vi "TCL.vi"() -> ()   [LabVIEW 2019]
uses:
  TPS Global.vi
panel:
  out "folder_base_2":path
  out "file_name_2":string
  out "file_basename_2":string
  out "time_string_2":string
  out "nfs_ok_2":bool
  out "nfs_ok":bool
  out "nfs_path":path
  out "signal_names":string[](array[string])
  out "time_string":string
  out "file_basename":string
  out "file_name":string
  out "folder_base":path
  in  "nfs_folder":string="z:\\e1039_data\\target_data\\NMR"
  out "discarded fragments":string[](array[string])
  out "signals":cluster{"name":string, "values":string[]}[](array[cluster])
  out "events (last 11)":string[][](array[string])
  out "fragments":string[](array[string])
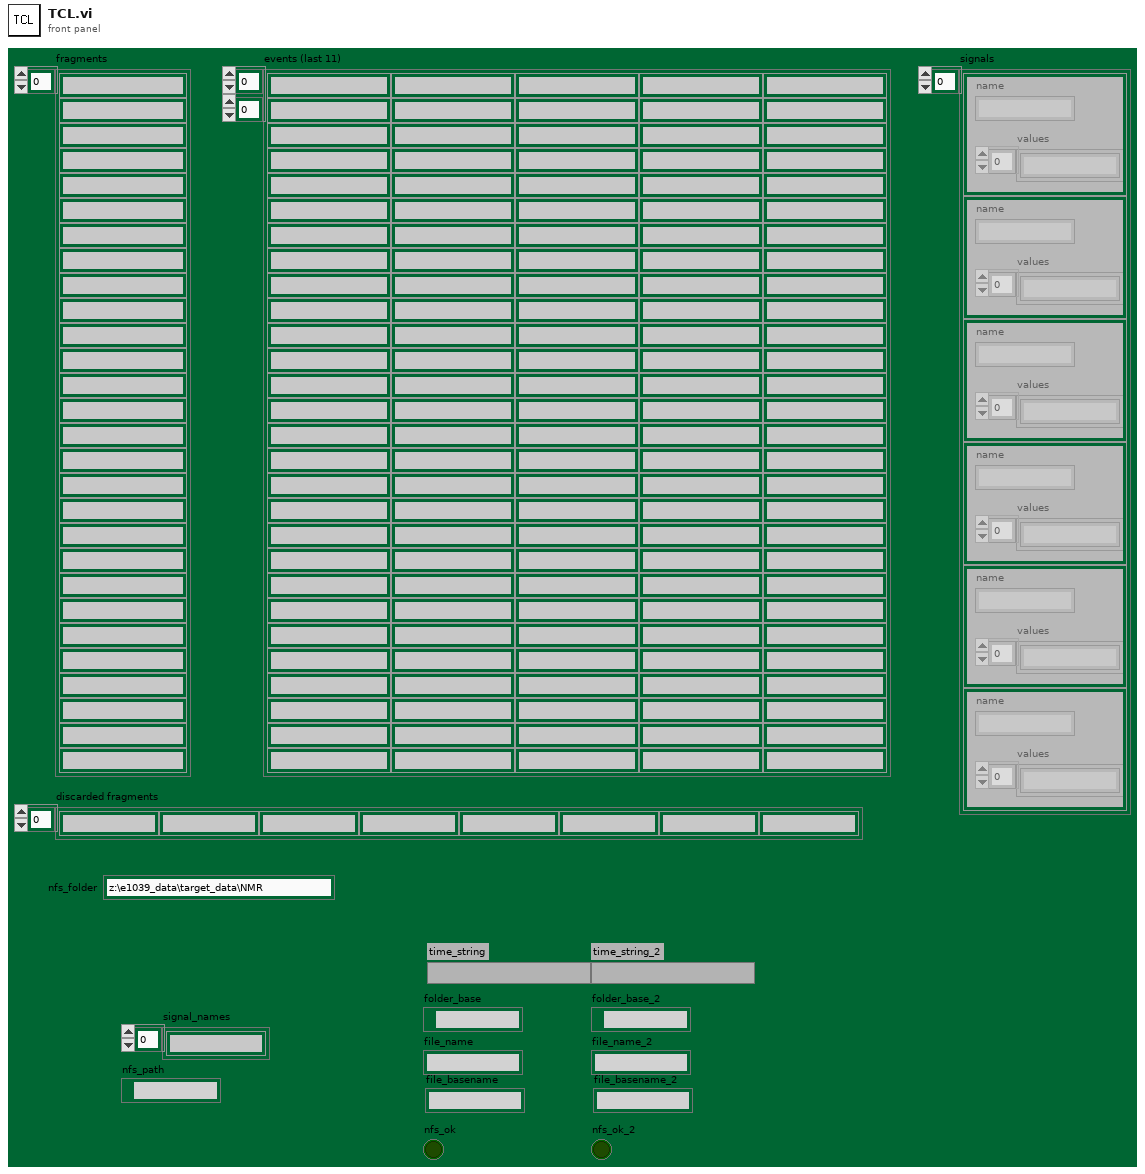
[diagram p1: front panel]
types:
  T1 = enum16{"open", "replace", "create", "open or create", "replace or create", "replace or create with confirmation"}
  T2 = enum16{"No Message", "Bad Message", "NewEventFile", "NewBaseFile", "Event=", "Ping=", "Address=", "Stop"}
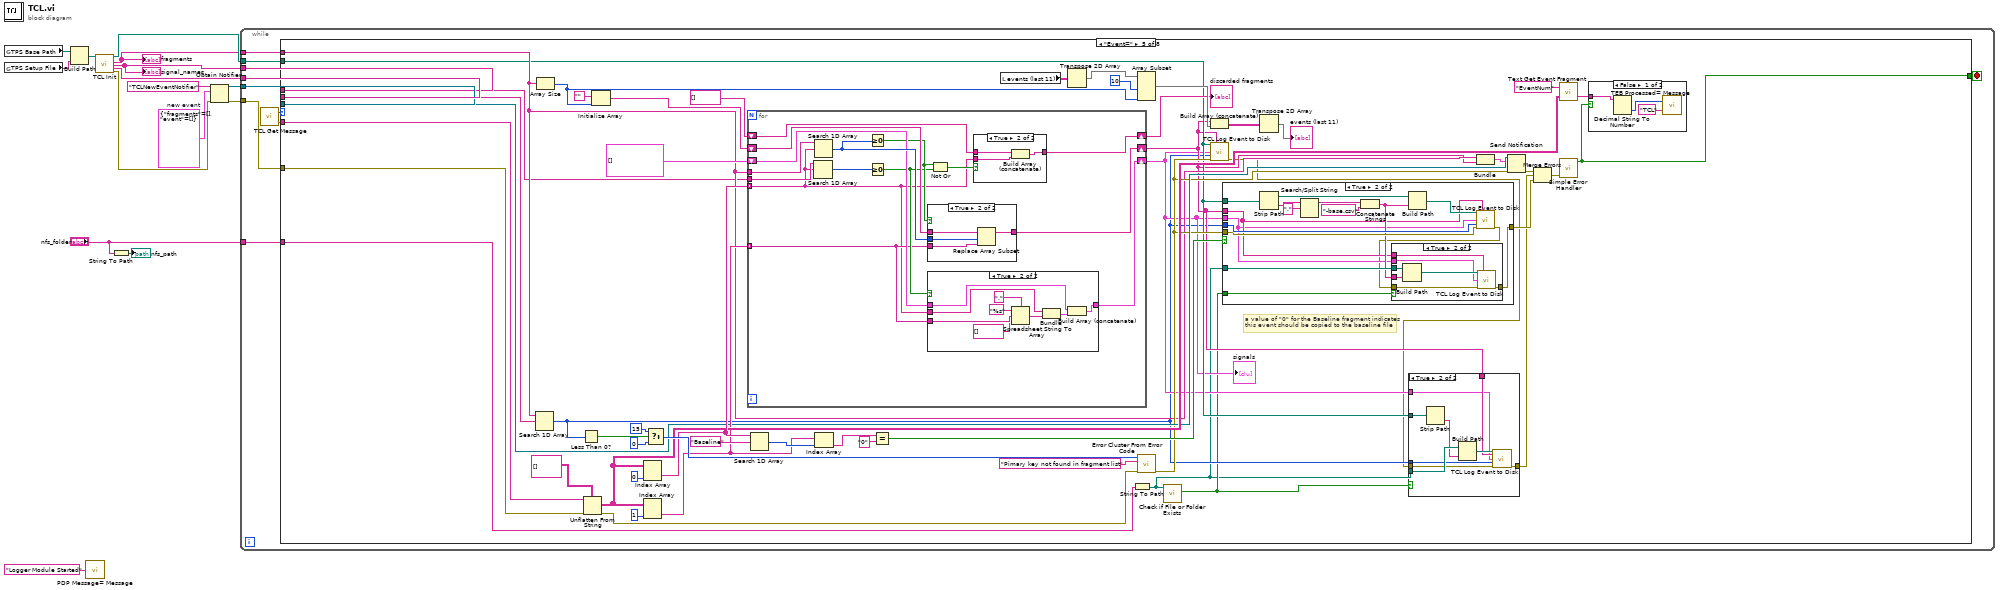
[diagram p0: block diagram]
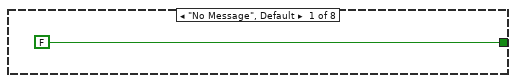
[diagram p2: hidden frame]
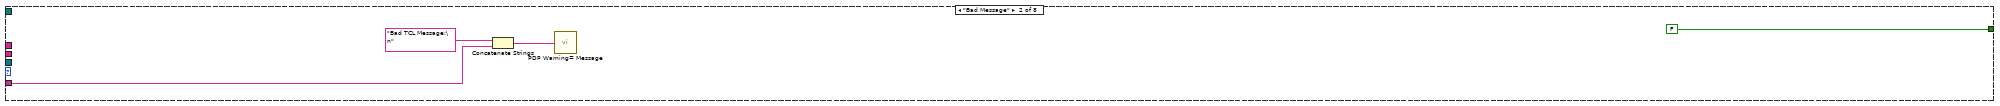
[diagram p3: hidden frame]
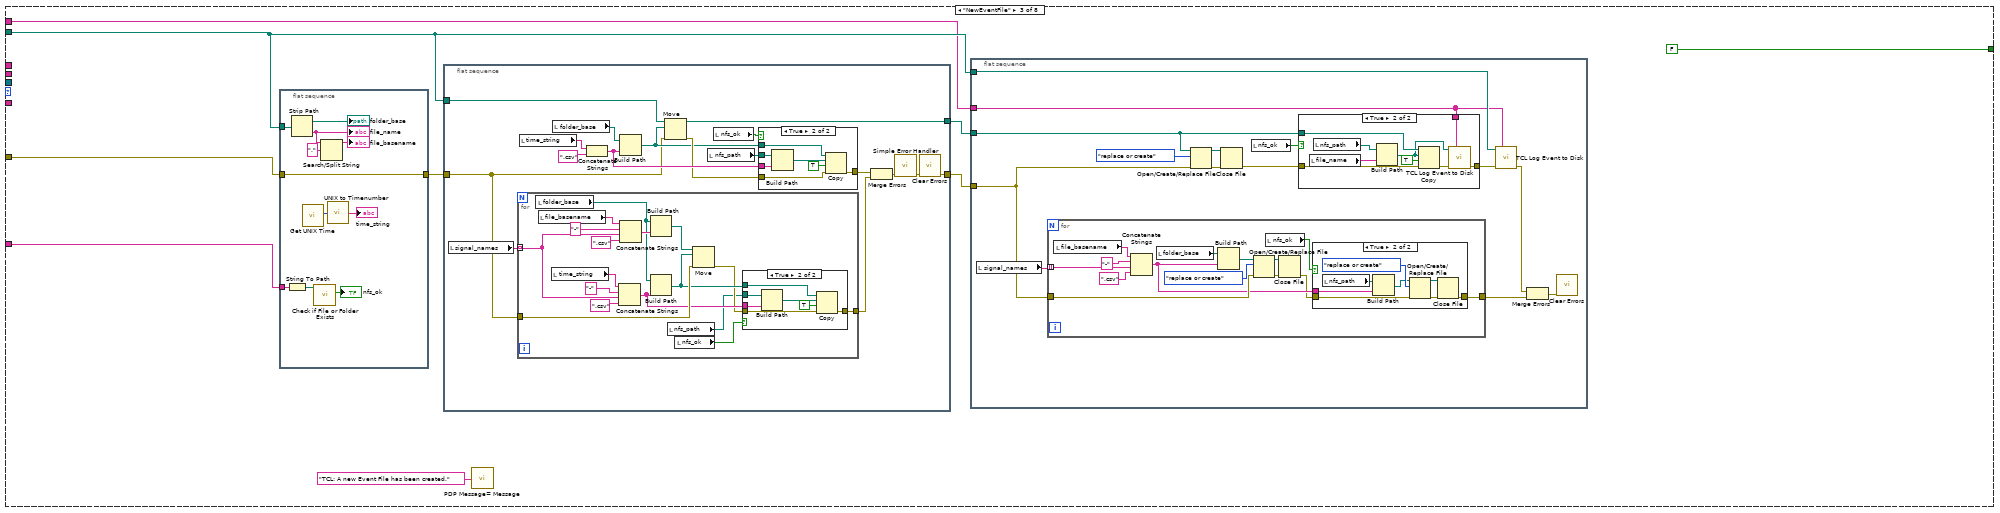
[diagram p4: hidden frame]
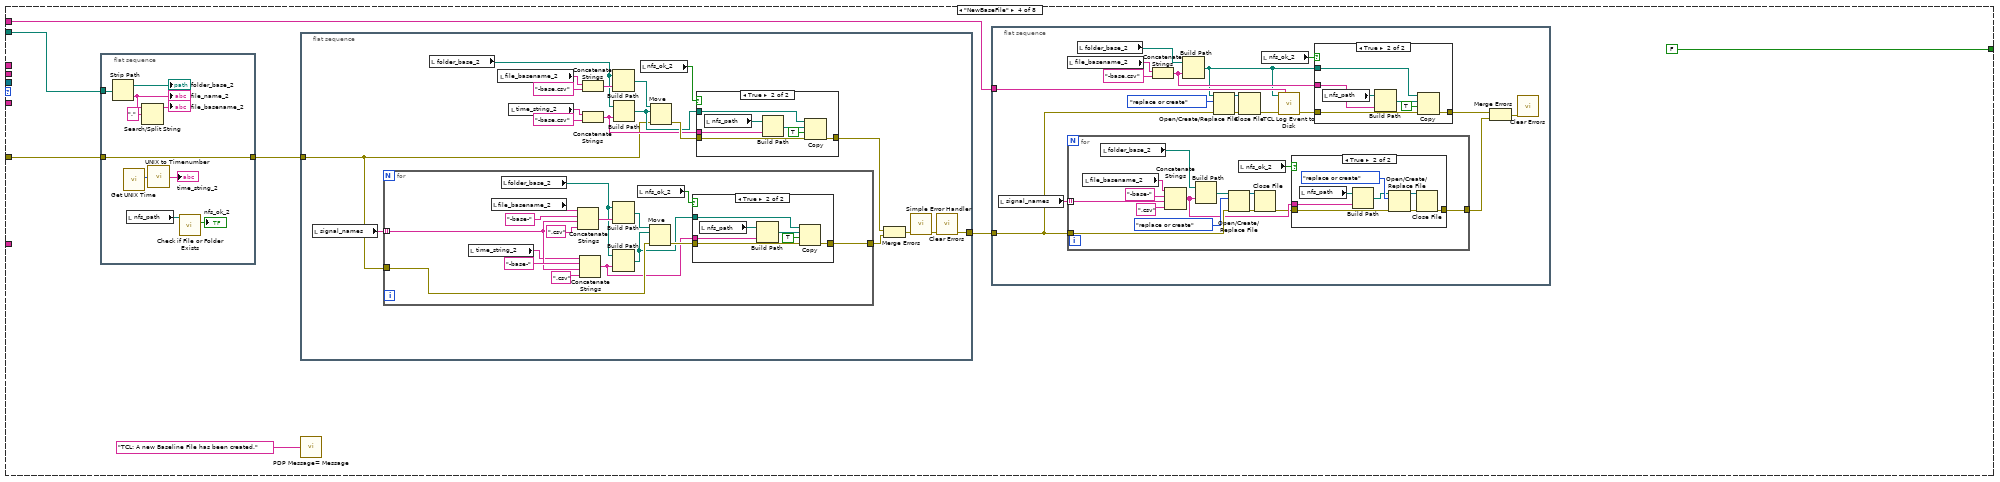
[diagram p9: hidden frame]
diagram:
  w6 = cluster{"fragments":string[], "event":string[]} {"fragments"=[], "event"=[]}  # new event
  n1 = global read "TPS Global.vi" "TPS Base Path"() -> (w14:path)
  n2 = global read "TPS Global.vi" "TPS Setup File"() -> (w13:string)
  n3 = Build Path(base path=w14, name or relative path=w13) -> (appended path=w12:path)
  n4 = call "PDP Message= Message.vi"("Message"="Logger Module Started") -> ()
  n5 = call "TCL Init.vi"("config file"=w12) -> ("event file"=w11:path, "fragments"=w9:string[], "signals"=w3:string[], "primary key"=w10:string, "error out"=w7:errorcluster)  [unwired: 14 in]
  "fragments" <- w9
  "signal_names" <- w3
  n6 = String To Path(string="nfs_folder") -> (path=→"nfs_path":path)
  n7 = Obtain Notifier(name (unnamed)="TCLNewEventNotifier", notification data type=w6, error in (no error)=w7) -> (notifier out=w4:refnum<notifier>, error out=w8:errorcluster)  [unwired: 1 in, 1 out]
  n8 = while {
    tunnel: w8 -> [w23]
    tunnel: w11 -> [w22]
    tunnel: w9 -> [w21]
    tunnel: w10 -> [w19]
    tunnel: w4 -> [w18]
    tunnel: "nfs_folder" -> [w17]
    tunnel: w3 -> [w16]
    stop <- w20 stop-if-true
    n9 = call "TCL Get Message.vi"() -> ("Text"=w24:string, "TCL Message Type"=w25:T2)
    n10 = case shown="\"Event=\"" w25 {
      tunnel: w24 -> [_ w28 _ _ w312 w387 w393 _]
      tunnel: w23 -> [_ _ w34 w148 w313 _ _ _]
      tunnel: w22 -> [_ _ w32 w149 w270 _ _ _]
      tunnel: w21 -> [_ _ w31 w151 w272 _ _ _]
      tunnel: [FALSE FALSE FALSE FALSE w278 FALSE FALSE TRUE] -> w20
      tunnel: w19 -> [_ _ _ _ w304 _ _ _]
      tunnel: w18 -> [_ _ _ _ w276 _ _ _]
      tunnel: w17 -> [_ _ w36 _ w271 _ _ _]
      tunnel: w16 -> [_ _ _ _ w264 _ _ _]
      frame "No Message", Default {
      }
      frame "Bad Message" {
        n11 = Concatenate Strings("Bad TCL Message:\n" ("Message"), w28) -> (w29:string)
        n12 = call "PDP Warning= Message.vi"("Message"=w29) -> ()
      }
      frame "NewEventFile" {
        n13 = flat-sequence {
          tunnel: w36 -> [w144]
          tunnel: w32 -> [w142]
          tunnel: w34 -> [w136]
          tunnel: [w136] -> w33
          frame #0 {
            n14 = String To Path(string=w144) -> (path=w137:path)
            n15 = Strip Path(path=w142) -> (stripped path=→"folder_base":path, name=w140:string)
            "file_name" <- w140
            n16 = call "Get UNIX Time.vi"() -> ("UNIX seconds"=w146:i32)  [unwired: 10 in, 1 out]
            n17 = call <vilib>:"Check if File or Folder Exists.vi"("path"=w137) -> ("file or folder exists?"=→"nfs_ok":bool)  [unwired: 8 in, 2 out]
            n18 = Search/Split String(string=w140, search string/char (-)=".") -> (substring before match=→"file_basename":string)  [unwired: 1 in, 2 out]
            n19 = call "UNIX to Timenumber.vi"("Seconds"=w146) -> ("Timestamp String"=→"time_string":string)
          }
        }
        n20 = flat-sequence {
          tunnel: [w98] -> w37
          tunnel: [w87] -> w35
          tunnel: w33 -> [w88]
          tunnel: w32 -> [w87]
          frame #0 {
            n21 = local read "signal_names"() -> (w93:string[])
            n22 = for {
              tunnel: w93 -> [w121] mode=indexing
              tunnel: w88 -> [w127]
              tunnel: [w116] -> w101
              n23 = local read "folder_base"() -> (w113:path)
              n24 = local read "file_basename"() -> (w114:string)
              n25 = local read "time_string"() -> (w115:string)
              n26 = Concatenate Strings(w115, "-" ("string"), w121, ".csv" ("string")) -> (w119:string)
              n27 = Concatenate Strings(w114, "-" ("string"), w121, ".csv" ("string")) -> (w126:string)
              n28 = Build Path(base path=w113, name or relative path=w126) -> (appended path=w123:path)
              n29 = Build Path(base path=w113, name or relative path=w119) -> (appended path=w118:path)
              n30 = local read "nfs_path"() -> (w111:path)
              n31 = local read "nfs_ok"() -> (w112:bool)
              n32 = Move(source path=w123, error in=w127, 10:w118) -> (error out=w117:errorcluster)  [unwired: 2 in, 2 out]
              n33 = case shown="True" w112 {
                tunnel: w111 -> [_ w135]
                tunnel: w119 -> [_ w134]
                tunnel: w118 -> [_ w132]
                tunnel: w117 -> [w128 w131]
                tunnel: [w128 w130] -> w116
                frame False {
                }
                frame True {
                  n34 = Build Path(base path=w135, name or relative path=w134) -> (appended path=w133:path)
                  n35 = Copy(8:w131, 9:TRUE ("overwrite (F)"), 10:w133, 11:w132) -> (0:w130:errorcluster)  [unwired: 1 in, 2 out]
                }
              }
            }
            n36 = local read "time_string"() -> (w91:string)
            n37 = local read "folder_base"() -> (w92:path)
            n38 = Concatenate Strings(w91, ".csv" ("string")) -> (w97:string)
            n39 = Build Path(base path=w92, name or relative path=w97) -> (appended path=w94:path)
            n40 = Move(source path=w87, error in=w88, 10:w94) -> (error out=w96:errorcluster)  [unwired: 2 in, 2 out]
            n41 = local read "nfs_path"() -> (w89:path)
            n42 = local read "nfs_ok"() -> (w90:bool)
            n43 = case shown="True" w90 {
              tunnel: w89 -> [_ w110]
              tunnel: w97 -> [_ w109]
              tunnel: w96 -> [w103 w108]
              tunnel: [w103 w107] -> w95
              tunnel: w94 -> [_ w105]
              frame False {
              }
              frame True {
                n44 = Build Path(base path=w110, name or relative path=w109) -> (appended path=w106:path)
                n45 = Copy(8:w108, 9:TRUE ("overwrite (F)"), 10:w106, 11:w105) -> (0:w107:errorcluster)  [unwired: 1 in, 2 out]
              }
            }
            n46 = Merge Errors(w95, w101) -> (w100:errorcluster)
            n47 = call <vilib>:"Simple Error Handler.vi"("error in (no error)"=w100) -> ("error out"=w99:errorcluster)  [unwired: 4 in, 4 out]
            n48 = call <vilib>:"Clear Errors.vi"("error in (no error)"=w99) -> ("error out"=w98:errorcluster)  [unwired: 5 in, 1 out]
          }
        }
        n49 = call "PDP Message= Message.vi"("Message"="TCL: A new Event File has been created.") -> ()
        n50 = flat-sequence {
          tunnel: w37 -> [w49]
          tunnel: w35 -> [w47]
          tunnel: w32 -> [w44]
          tunnel: w31 -> [w40]
          frame #0 {
            n51 = local read "signal_names"() -> (w46:string[])
            n52 = for {
              tunnel: w46 -> [w76] mode=indexing
              tunnel: w49 -> [w74]
              tunnel: [w68] -> w50
              n53 = local read "file_basename"() -> (w65:string)
              n54 = Concatenate Strings(w65, "-" ("string"), w76, ".csv" ("string")) -> (w70:string)
              n55 = local read "folder_base"() -> (w66:path)
              n56 = Build Path(base path=w66, name or relative path=w70) -> (appended path=w75:path)
              n57 = Open/Create/Replace File(file path (use dialog)=w75, error in=w74, operation (0:open)=T1."replace or create") -> (refnum out=w72:refnum<file>, error out=w71:errorcluster)  [unwired: 3 in, 1 out]
              n58 = local read "nfs_ok"() -> (w67:bool)
              n59 = Close File(refnum=w72, error in=w71) -> (error out=w69:errorcluster)  [unwired: 1 out]
              n60 = case shown="True" w67 {
                tunnel: w70 -> [_ w86]
                tunnel: w69 -> [w78 w82]
                tunnel: [w78 w83] -> w68
                frame False {
                }
                frame True {
                  n61 = local read "nfs_path"() -> (w79:path)
                  n62 = Build Path(base path=w79, name or relative path=w86) -> (appended path=w80:path)
                  n63 = Open/Create/Replace File(file path (use dialog)=w80, error in=w82, operation (0:open)=T1."replace or create") -> (refnum out=w85:refnum<file>, error out=w84:errorcluster)  [unwired: 3 in, 1 out]
                  n64 = Close File(refnum=w85, error in=w84) -> (error out=w83:errorcluster)  [unwired: 1 out]
                }
              }
            }
            n65 = Open/Create/Replace File(file path (use dialog)=w47, error in=w49, operation (0:open)=T1."replace or create") -> (refnum out=w52:refnum<file>, error out=w51:errorcluster)  [unwired: 3 in, 1 out]
            n66 = Close File(refnum=w52, error in=w51) -> (error out=w48:errorcluster)  [unwired: 1 out]
            n67 = local read "nfs_ok"() -> (w45:bool)
            n68 = case shown="True" w45 {
              tunnel: w48 -> [w54 w63]
              tunnel: [w54 w60] -> w43
              tunnel: w47 -> [_ w62]
              tunnel: w40 -> [_ w58]
              frame False {
              }
              frame True {
                n69 = local read "file_name"() -> (w55:string)
                n70 = local read "nfs_path"() -> (w56:path)
                n71 = Build Path(base path=w56, name or relative path=w55) -> (appended path=w59:path)
                n72 = Copy(8:w63, 9:TRUE ("overwrite (F)"), 10:w59, 11:w62) -> (0:w61:errorcluster)  [unwired: 1 in, 2 out]
                n73 = call "TCL Log Event to Disk.vi"("event file"=w59, "event"=w58, "error in (no error)"=w61) -> ("error out"=w60:errorcluster)  [unwired: 12 in]
              }
            }
            n74 = call "TCL Log Event to Disk.vi"("event file"=w44, "event"=w40, "error in (no error)"=w43) -> ("error out"=w42:errorcluster)  [unwired: 12 in]
            n75 = Merge Errors(w42, w50) -> (w41:errorcluster)
            n76 = call <vilib>:"Clear Errors.vi"("error in (no error)"=w41) -> ()  [unwired: 5 in, 2 out]
          }
        }
      }
      frame "NewBaseFile" {
        n77 = flat-sequence {
          tunnel: w149 -> [w258]
          tunnel: w148 -> [w252]
          tunnel: [w252] -> w147
          frame #0 {
            n78 = Strip Path(path=w258) -> (stripped path=→"folder_base_2":path, name=w256:string)
            "file_name_2" <- w256
            n79 = call "Get UNIX Time.vi"() -> ("UNIX seconds"=w261:i32)  [unwired: 10 in, 1 out]
            n80 = local read "nfs_path"() -> (w253:path)
            n81 = Search/Split String(string=w256, search string/char (-)=".") -> (substring before match=→"file_basename_2":string)  [unwired: 1 in, 2 out]
            n82 = call "UNIX to Timenumber.vi"("Seconds"=w261) -> ("Timestamp String"=→"time_string_2":string)
            n83 = call <vilib>:"Check if File or Folder Exists.vi"("path"=w253) -> ("file or folder exists?"=→"nfs_ok_2":bool)  [unwired: 8 in, 2 out]
          }
        }
        n84 = flat-sequence {
          tunnel: [w212] -> w150
          tunnel: w147 -> [w203]
          frame #0 {
            n85 = local read "signal_names"() -> (w211:string[])
            n86 = for {
              tunnel: w211 -> [w237] mode=indexing
              tunnel: w203 -> [w243]
              tunnel: [w231] -> w216
              n87 = local read "time_string_2"() -> (w235:string)
              n88 = local read "file_basename_2"() -> (w233:string)
              n89 = local read "folder_base_2"() -> (w234:path)
              n90 = Concatenate Strings(w233, "-base-" ("string"), w237, ".csv" ("string")) -> (w242:string)
              n91 = Concatenate Strings(w235, "-base-" ("string"), w237, ".csv" ("string")) -> (w229:string)
              n92 = Build Path(base path=w234, name or relative path=w242) -> (appended path=w239:path)
              n93 = Build Path(base path=w234, name or relative path=w229) -> (appended path=w228:path)
              n94 = local read "nfs_ok_2"() -> (w230:bool)
              n95 = Move(source path=w239, error in=w243, 10:w228) -> (error out=w232:errorcluster)  [unwired: 2 in, 2 out]
              n96 = case shown="True" w230 {
                tunnel: w229 -> [_ w251]
                tunnel: w228 -> [_ w249]
                tunnel: w232 -> [w244 w248]
                tunnel: [w244 w247] -> w231
                frame False {
                }
                frame True {
                  n97 = local read "nfs_path"() -> (w245:path)
                  n98 = Build Path(base path=w245, name or relative path=w251) -> (appended path=w250:path)
                  n99 = Copy(8:w248, 9:TRUE ("overwrite (F)"), 10:w250, 11:w249) -> (0:w247:errorcluster)  [unwired: 1 in, 2 out]
                }
              }
            }
            n100 = local read "folder_base_2"() -> (w208:path)
            n101 = local read "file_basename_2"() -> (w209:string)
            n102 = local read "time_string_2"() -> (w210:string)
            n103 = Concatenate Strings(w209, "-base.csv" ("string")) -> (w218:string)
            n104 = Concatenate Strings(w210, "-base.csv" ("string")) -> (w205:string)
            n105 = Build Path(base path=w208, name or relative path=w218) -> (appended path=w215:path)
            n106 = Build Path(base path=w208, name or relative path=w205) -> (appended path=w204:path)
            n107 = local read "nfs_ok_2"() -> (w202:bool)
            n108 = Move(source path=w215, error in=w203, 10:w204) -> (error out=w207:errorcluster)  [unwired: 2 in, 2 out]
            n109 = case shown="True" w202 {
              tunnel: w205 -> [_ w227]
              tunnel: w204 -> [_ w225]
              tunnel: w207 -> [w220 w224]
              tunnel: [w220 w223] -> w206
              frame False {
              }
              frame True {
                n110 = local read "nfs_path"() -> (w221:path)
                n111 = Build Path(base path=w221, name or relative path=w227) -> (appended path=w226:path)
                n112 = Copy(8:w224, 9:TRUE ("overwrite (F)"), 10:w226, 11:w225) -> (0:w223:errorcluster)  [unwired: 1 in, 2 out]
              }
            }
            n113 = Merge Errors(w206, w216) -> (w214:errorcluster)
            n114 = call <vilib>:"Simple Error Handler.vi"("error in (no error)"=w214) -> ("error out"=w213:errorcluster)  [unwired: 4 in, 4 out]
            n115 = call <vilib>:"Clear Errors.vi"("error in (no error)"=w213) -> ("error out"=w212:errorcluster)  [unwired: 5 in, 1 out]
          }
        }
        n116 = call "PDP Message= Message.vi"("Message"="TCL: A new Baseline File has been created.") -> ()
        n117 = flat-sequence {
          tunnel: w151 -> [w166]
          tunnel: w150 -> [w164]
          frame #0 {
            n118 = local read "signal_names"() -> (w161:string[])
            n119 = local read "file_basename_2"() -> (w162:string)
            n120 = for {
              tunnel: w161 -> [w190] mode=indexing
              tunnel: w164 -> [w188]
              tunnel: [w179] -> w167
              n121 = local read "file_basename_2"() -> (w183:string)
              n122 = local read "folder_base_2"() -> (w184:path)
              n123 = Concatenate Strings(w183, "-base-" ("string"), w190, ".csv" ("string")) -> (w181:string)
              n124 = Build Path(base path=w184, name or relative path=w181) -> (appended path=w189:path)
              n125 = Open/Create/Replace File(file path (use dialog)=w189, error in=w188, operation (0:open)=T1."replace or create") -> (refnum out=w186:refnum<file>, error out=w185:errorcluster)  [unwired: 3 in, 1 out]
              n126 = local read "nfs_ok_2"() -> (w182:bool)
              n127 = Close File(refnum=w186, error in=w185) -> (error out=w180:errorcluster)  [unwired: 1 out]
              n128 = case shown="True" w182 {
                tunnel: w181 -> [_ w201]
                tunnel: w180 -> [w193 w197]
                tunnel: [w193 w198] -> w179
                frame False {
                }
                frame True {
                  n129 = local read "nfs_path"() -> (w194:path)
                  n130 = Build Path(base path=w194, name or relative path=w201) -> (appended path=w195:path)
                  n131 = Open/Create/Replace File(file path (use dialog)=w195, error in=w197, operation (0:open)=T1."replace or create") -> (refnum out=w200:refnum<file>, error out=w199:errorcluster)  [unwired: 3 in, 1 out]
                  n132 = Close File(refnum=w200, error in=w199) -> (error out=w198:errorcluster)  [unwired: 1 out]
                }
              }
            }
            n133 = local read "folder_base_2"() -> (w163:path)
            n134 = Concatenate Strings(w162, "-base.csv" ("string")) -> (w156:string)
            n135 = Build Path(base path=w163, name or relative path=w156) -> (appended path=w155:path)
            n136 = Open/Create/Replace File(file path (use dialog)=w155, error in=w164, operation (0:open)=T1."replace or create") -> (refnum out=w169:refnum<file>, error out=w168:errorcluster)  [unwired: 3 in, 1 out]
            n137 = Close File(refnum=w169, error in=w168) -> (error out=w160:errorcluster)  [unwired: 1 out]
            n138 = local read "nfs_ok_2"() -> (w159:bool)
            n139 = call "TCL Log Event to Disk.vi"("event file"=w155, "event"=w166, "error in (no error)"=w160) -> ("error out"=w158:errorcluster)  [unwired: 12 in]
            n140 = case shown="True" w159 {
              tunnel: w158 -> [w171 w177]
              tunnel: [w171 w176] -> w157
              tunnel: w156 -> [_ w174]
              tunnel: w155 -> [_ w172]
              frame False {
              }
              frame True {
                n141 = local read "nfs_path"() -> (w178:path)
                n142 = Build Path(base path=w178, name or relative path=w174) -> (appended path=w173:path)
                n143 = Copy(8:w177, 9:TRUE ("overwrite (F)"), 10:w173, 11:w172) -> (0:w176:errorcluster)  [unwired: 1 in, 2 out]
              }
            }
            n144 = Merge Errors(w157, w167) -> (w154:errorcluster)
            n145 = call <vilib>:"Clear Errors.vi"("error in (no error)"=w154) -> ()  [unwired: 5 in, 2 out]
          }
        }
      }
      frame "Event=" {
        # "a value of \"0\" for the Baseline fragment indicates\nthis event should be copied to the baseline file"
        n146 = Search 1D Array(1D array=w272, element=w304) -> (index of element=w267:i32)  [unwired: 1 in]
        n147 = Array Size(array=w272) -> (size(s)=w283:i32)
        n148 = Less Than 0?(x=w267) -> (x < 0?=w301:bool)
        n149 = Unflatten From String(type=string[][] [], binary string=w312, error in (no error)=w313) -> (value=w287:string[][], error out=w303:errorcluster)  [unwired: 2 in, 1 out]
        n150 = Initialize Array("", w283) -> (w308:string[])
        n151 = Index Array(array=w287, index (col)=0) -> (element=w297:string[])  [unwired: 1 in]
        n152 = Index Array(array=w287, index (col)=1) -> (element=w277:string[])  [unwired: 1 in]
        n153 = Select(t=15, s=w301, f=0) -> (s? t:f=w300:i32)
        n154 = for {
          tunnel: w297 -> [w352] mode=indexing
          tunnel: w277 -> [w354] mode=indexing
          tunnel: w272 -> [w366]
          tunnel: w264 -> [w365]
          shift-right: [w362] -> w269
          shift-left: w308 -> [w363]
          shift-right: [w353] -> w281
          shift-left: string[] [] -> [w355]
          shift-right: [w359] -> w268
          shift-left: cluster{"name":string, "values":string[]}[] [] ("signals") -> [w360]
          n155 = Search 1D Array(1D array=w365, element=w352) -> (index of element=w361:i32)  [unwired: 1 in]
          n156 = Search 1D Array(1D array=w366, element=w352) -> (index of element=w364:i32)  [unwired: 1 in]
          n157 = Greater Or Equal To 0?(x=w364) -> (x >= 0?=w358:bool)
          n158 = Greater Or Equal To 0?(x=w361) -> (x >= 0?=w357:bool)
          n159 = case shown="True" w358 {
            tunnel: w364 -> [_ w385]
            tunnel: w354 -> [_ w384]
            tunnel: w363 -> [w381 w383]
            tunnel: [w381 w382] -> w362
            frame False {
            }
            frame True {
              n160 = Replace Array Subset(array=w383, new element=w384, index=w385) -> (w382:string[])
            }
          }
          n161 = case shown="True" w357 {
            tunnel: w360 -> [w371 w380]
            tunnel: w352 -> [_ w378]
            tunnel: w354 -> [_ w375]
            tunnel: [w371 w372] -> w359
            frame False {
            }
            frame True {
              n162 = Spreadsheet String To Array(delimiter (Tab)=",", format string="%s", spreadsheet string=w375, array type (2D Dbl)=string[] []) -> (array=w374:string[])
              n163 = Bundle(w378, w374) -> (w379:cluster{string, string[]})  [unwired: 1 in]
              n164 = Build Array (concatenate)(w380, w379) -> (w372:cluster{"name":string, "values":string[]}[])
            }
          }
          n165 = Not Or(1:w357, 2:w358) -> (0:w356:bool)
          n166 = case shown="True" w356 {
            tunnel: w355 -> [w367 w370]
            tunnel: w352 -> [_ w369]
            tunnel: [w367 w368] -> w353
            frame False {
            }
            frame True {
              n167 = Build Array (concatenate)(w370, w369) -> (w368:string[])
            }
          }
        }
        "discarded fragments" <- w281
        "signals" <- w268
        n168 = Search 1D Array(1D array=w297, element="Baseline") -> (index of element=w295:i32)  [unwired: 1 in]
        n169 = Index Array(array=w277, index=w295) -> (element=w294:string)
        n170 = Equal?(x=w294, y="0") -> (x = y?=w292:bool)
        n171 = local read "events (last 11)"() -> (w279:string[][])
        n172 = Transpose 2D Array(2D array=w279) -> (transposed array=w282:string[][])
        n173 = String To Path(string=w271) -> (path=w262:path)
        n174 = Array Subset(array=w282, length (row)=10, length (col)=w283) -> (w284:string[][])  [unwired: 2 in]
        n175 = call <vilib>:"Error Cluster From Error Code.vi"("error in (no error)"=w303, "error message (\"\")"="Pimary key not found in fragment list" ("error message (\"\")"), "error code (0)"=w300) -> ("error out"=w275:errorcluster)  [unwired: 6 in]
        n176 = call <vilib>:"Check if File or Folder Exists.vi"("path"=w262) -> ("file or folder exists?"=w263:bool)  [unwired: 8 in, 2 out]
        n177 = Build Array (concatenate)(w269, w284) -> (w285:string[][])
        n178 = call "TCL Log Event to Disk.vi"("event file"=w270, "event"=w269, "signals"=w268, "primary key"=w267, "error in (no error)"=w275) -> ("error out"=w265:errorcluster)  [unwired: 10 in]
        n179 = case shown="True" w292 {
          tunnel: w269 -> [_ w331]
          tunnel: w270 -> [_ w343]
          tunnel: w268 -> [_ w330]
          tunnel: w267 -> [_ w341]
          tunnel: w275 -> [w327 w340]
          tunnel: [w327 w329] -> w291
          tunnel: w263 -> [_ w334]
          tunnel: w262 -> [_ w333]
          frame False {
          }
          frame True {
            n180 = Strip Path(path=w343) -> (stripped path=w336:path, name=w339:string)
            n181 = Search/Split String(string=w339, search string/char (-)=".") -> (substring before match=w337:string)  [unwired: 1 in, 2 out]
            n182 = Concatenate Strings(w337, "-base.csv" ("string")) -> (w332:string)
            n183 = Build Path(base path=w336, name or relative path=w332) -> (appended path=w335:path)
            n184 = call "TCL Log Event to Disk.vi"("event file"=w335, "event"=w331, "signals"=w330, "primary key"=w341, "error in (no error)"=w340) -> ("error out"=w328:errorcluster)  [unwired: 10 in]
            n185 = case shown="True" w334 {
              tunnel: w333 -> [_ w351]
              tunnel: w332 -> [_ w350]
              tunnel: w331 -> [_ w348]
              tunnel: w330 -> [_ w347]
              tunnel: [w344 w346] -> w329
              tunnel: w328 -> [w344 w345]
              frame False {
              }
              frame True {
                n186 = Build Path(base path=w351, name or relative path=w350) -> (appended path=w349:path)
                n187 = call "TCL Log Event to Disk.vi"("event file"=w349, "event"=w348, "signals"=w347, "error in (no error)"=w345) -> ("error out"=w346:errorcluster)  [unwired: 11 in]
              }
            }
          }
        }
        n188 = Transpose 2D Array(2D array=w285) -> (transposed array=→"events (last 11)":string[][])
        n189 = case shown="True" w263 {
          tunnel: w262 -> [_ w322]
          tunnel: w270 -> [_ w323]
          tunnel: w269 -> [_ w319]
          tunnel: w268 -> [_ w318]
          tunnel: w267 -> [_ w317]
          tunnel: w265 -> [w314 w316]
          tunnel: [w314 w315] -> w266
          frame False {
          }
          frame True {
            n190 = Strip Path(path=w323) -> (name=w321:string)  [unwired: 1 out]
            n191 = Build Path(base path=w322, name or relative path=w321) -> (appended path=w320:path)
            n192 = call "TCL Log Event to Disk.vi"("event file"=w320, "event"=w319, "signals"=w318, "primary key"=w317, "error in (no error)"=w316) -> ("error out"=w315:errorcluster)  [unwired: 10 in]
          }
        }
        n193 = Bundle("fragments"=w272, w269) -> (w273:cluster{"fragments":string[], string[]})  [unwired: 1 in]
        n194 = Send Notification(notification=w273, notifier=w276, error in (no error)=w275) -> (error out=w274:errorcluster)  [unwired: 1 out]
        n195 = Merge Errors(w274, w266, w291) -> (w290:errorcluster)
        n196 = call "Text Get Event Fragment.vi"("Event"=w287, "Fragment Type"="EventNum") -> ("Fragment"=w288:string)  [unwired: 1 out]
        n197 = call <vilib>:"Simple Error Handler.vi"("error in (no error)"=w290) -> ("error?"=w278:bool)  [unwired: 4 in, 4 out]
        n198 = case shown="False" w278 {
          tunnel: w288 -> [w324 _]
          frame False {
            n199 = Decimal String To Number(string=w324) -> (number=w325:i32)  [unwired: 2 in, 1 out]
            n200 = call "TEB Processed= Message.vi"("Module Name"="TCL", "Event Number"=w325) -> ()
          }
          frame True {
          }
        }
      }
      frame "Ping=" {
        n201 = Get Date/Time In Seconds() -> (seconds since 1Jan1904=w388:timestamp)
        n202 = To Double Precision Float(number=w388) -> (double precision float=w390:dbl)
        n203 = Format Into String(format string="PingResponse=TCL,%.0f", w390) -> (resulting string=w389:string)  [unwired: 2 in, 1 out]
        n204 = call "Message Send.vi"("Message"=w389, "Destination"=w387) -> ()
      }
      frame "Address=" {
        n205 = Scan From String(format string="%3s,%[.0-9]:%d" ("Format String"), input string=w393) -> (output 1=w395:string, output 2=w396:string, output 3=w394:i32)  [unwired: 5 in, 3 out]
        n206 = call "Message Set Module Address.vi"("Port"=w394, "Address"=w396, "Module"=w395) -> ()
      }
      frame "Stop" {
      }
    }
  }
